vi "RS232_Write.vi"(8 "错误输入（无错误）":errorcluster, 9 "写入缓冲区":string, 11 "VISA资源名称":refnum<visa-resource-name>) -> (0 "错误输出":errorcluster, 3 "VISA资源名称输出":refnum<visa-resource-name>)   [LabVIEW 2018]
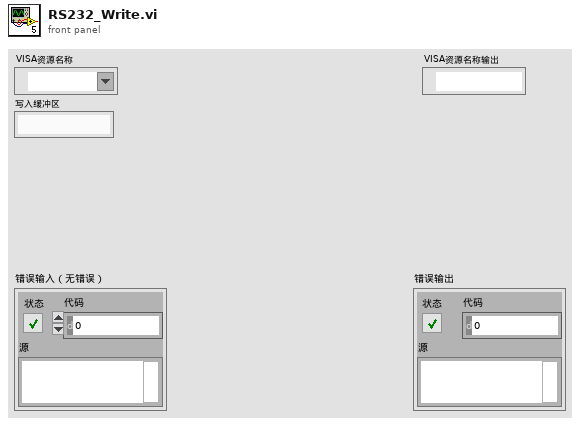
[diagram p1: front panel]
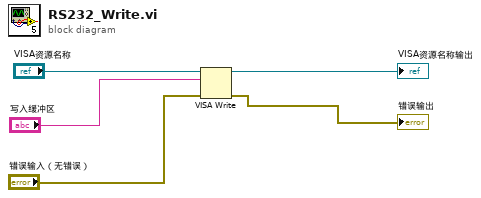
[diagram p0: block diagram]
diagram:
  n1 = VISA Write(VISA resource name="VISA资源名称", write buffer="写入缓冲区", error in (no error)="错误输入（无错误）") -> (VISA resource name out=→"VISA资源名称输出":refnum<visa-resource-name>, error out=→"错误输出":errorcluster)  [unwired: 1 out]
